vi "Read Valid Pixels Size.vi"(8 "error in (no error)":errorcluster, 11 "Image Undistorter in":refnum<class "Image Undistorter.lvclass">) -> (0 "error out":errorcluster, 2 "Image Size":T1, 3 "Image Undistorter":refnum<class "Image Undistorter.lvclass">)   [LabVIEW 2020, in "image.lvlib" / "Image Undistorter.lvclass"]
doc: "Get the size of the undistored image valid-pixel region."
uses:
  Image Undistorter.lvclass
  Image Undistorter.lvclass/Image Undistorter.ctl
  common/Image Size (Integer).ctl
  common/common.lvlib
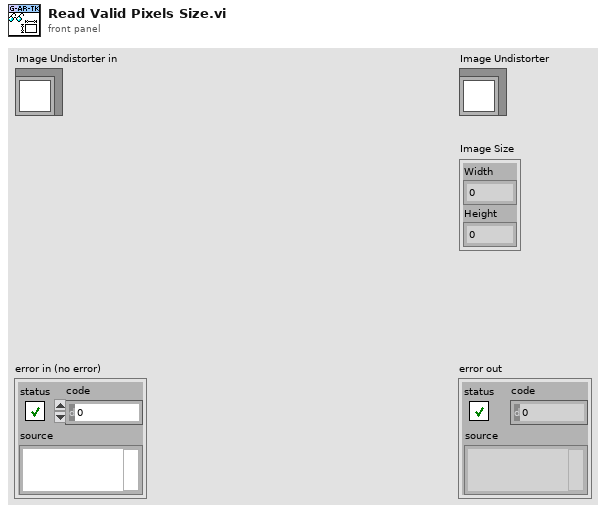
[diagram p1: front panel]
types:
  T1 = typedef "common.lvlib/Image Size (Integer).ctl" = cluster{"Width":u16, "Height":u16}
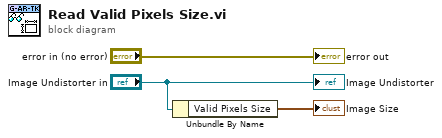
[diagram p0: block diagram]
diagram:
  n1 = Unbundle By Name("Image Undistorter in") -> ("Valid Pixels Size"=→"Image Size":T1)
  "error out" <- "error in (no error)"
  "Image Undistorter" <- "Image Undistorter in"
